vi "GetLimsTestsForBench.vi"(8 "error in (no error)":errorcluster, 9 "creation date":timestamp, 10 "workbench":string, 11 "ByteGSAPIBase in":refnum<class "ByteGSAPIBase.lvclass">) -> (0 "error out":errorcluster, 2 "list of tests":T1[](array[typedef]), 3 "ByteGSAPIBase out":refnum<class "ByteGSAPIBase.lvclass">)   [LabVIEW 2019, in "ByteGSWebAPI.lvlib" / "ByteGSAPIBase.lvclass"]
doc: "Request the list of Tests based on Workstation and Creation date (optional)"
uses:
  ByteGSAPIBase.lvclass
  TypeDef/Test.ctl
  TypeDef/Asset.ctl
  ByteGSAPIBase.lvclass/ByteGSAPIBase.ctl
  <vilib>/Bytelabs/ByteREST/ByteRESTClass/ByteRESTBase/RESTBase.lvclass
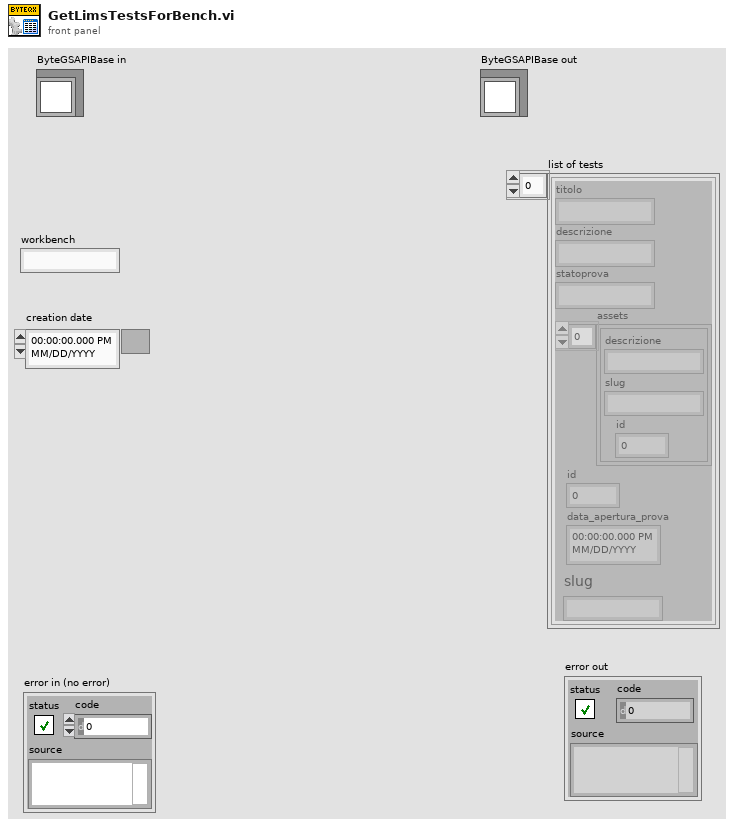
[diagram p1: front panel]
types:
  T1 = typedef "ByteGSWebAPI.lvlib/ByteGSAPIBase.lvclass/Test.ctl" = cluster{"titolo":string, "descrizione":string, "statoprova":string, "assets":T2[], "id":i32, "data_apertura_prova":timestamp, "slug":string}
  T2 = typedef "ByteGSWebAPI.lvlib/ByteGSAPIBase.lvclass/Asset.ctl" = cluster{"descrizione":string, "slug":string, "id":i32}
  T3 = cluster{"titolo":string, "descrizione":string, "statoprova":string, "assets":cluster{"descrizione":string, "slug":string, "id":i32}[], "data_apertura_prova":string, "id":i32, "slug":string}[]
  T4 = cluster{"descrizione":string, "slug":string, "id":i32}[]
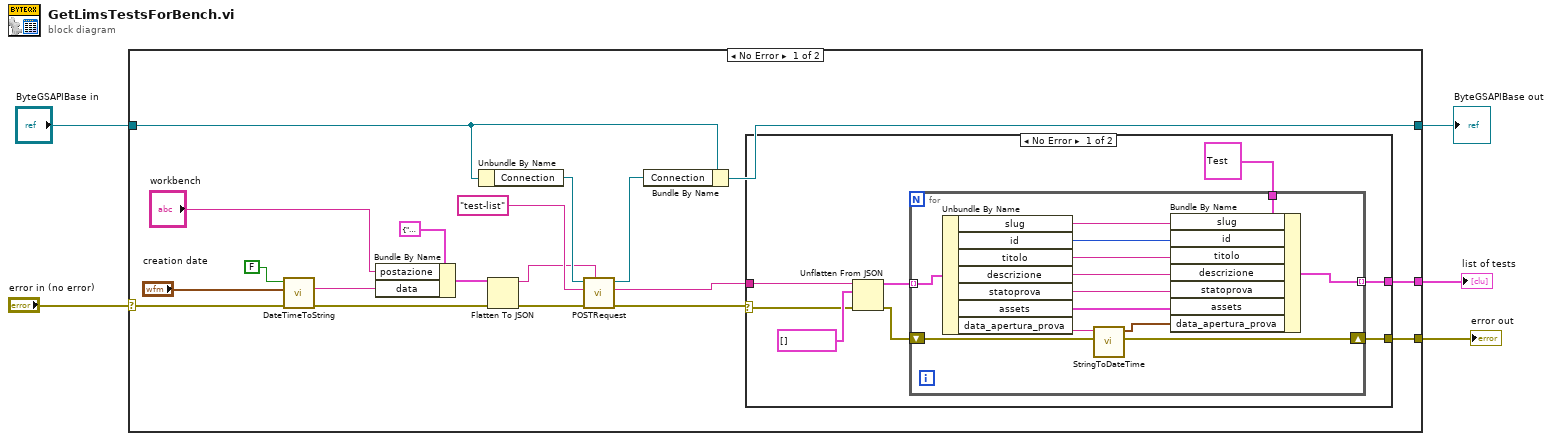
[diagram p0: block diagram]
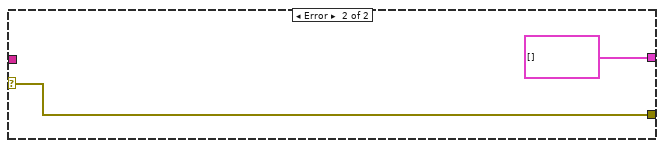
[diagram p2: hidden frame]
diagram:
  n1 = case shown="No Error" "error in (no error)" {
    selector: "error in (no error)" -> [w11 w49]
    tunnel: [w17 w49] -> w4
    tunnel: [w22 w48] -> w2
    tunnel: "ByteGSAPIBase in" -> [w15 w48]
    tunnel: [w16 _] -> w1
    frame No Error {
      n2 = call "DateTimeToString.vi"("error in"=w11, "current time"="creation date", "include Time?"=FALSE ("Time")) -> ("error out"=w12:errorcluster, "date string"=w10:string)  [unwired: 7 in]
      n3 = Bundle By Name(cluster=cluster{"postazione":string, "data":string} {"postazione"="", "data"=""} ("Request"), "postazione"="workbench", "data"=w10) -> (w13:cluster{"postazione":string, "data":string})
      n4 = Unbundle By Name(w15) -> ("Connection"=w24:refnum<class "RESTBase.lvclass">)
      n5 = Flatten To JSON(anything=w13, error in (no error)=w12) -> (JSON string=w20:string, 11:w19:errorcluster)  [unwired: 1 in]
      n6 = call-dynamic "POSTRequest.vi"("Body in"=w20, "error in (no error)"=w19, "Request"="test-list", "ByteRESTBase in"=w24) -> ("error out"=w7:errorcluster, "Body"=w18:string, "ByteRESTBase out"=w23:refnum<class "RESTBase.lvclass">)  [unwired: 4 in, 1 out]
      n7 = Bundle By Name(cluster=w15, "Connection"=w23) -> (w22:refnum<class "ByteGSAPIBase.lvclass">)
      n8 = case shown="No Error" w7 {
        selector: w7 -> [w25 w47]
        tunnel: w18 -> [w32 _]
        tunnel: [w28 w47] -> w17
        tunnel: [w27 T1[] []] -> w16
        frame No Error {
          n9 = Unflatten From JSON(JSON string=w32, type and defaults=T3 [], error in (no error)=w25) -> (value=w30:T3, error out=w29:errorcluster)  [unwired: 4 in]
          n10 = for {
            tunnel: w30 -> [w45] mode=indexing
            tunnel: T1 {"titolo"="", "descrizione"="", "statoprova"="", "assets"=[], "id"=0, "data_apertura_prova"=timestamp(0 s since 1904-01-01), "slug"=""} ("ByteGSWebAPI.lvlib:ByteGSAPIBase.lvclass:Test") -> [w44]
            shift-right: [w34] -> w28
            shift-left: w29 -> [w35]
            tunnel: [w38] -> w27 mode=indexing
            n11 = Unbundle By Name(w45) -> ("slug"=w33:string, "id"=w43:i32, "titolo"=w42:string, "descrizione"=w41:string, "statoprova"=w40:string, "assets"=w39:T4, "data_apertura_prova"=w37:string)
            n12 = call "StringToDateTime.vi"("error in (no error)"=w35, "datetime string"=w37) -> ("error out"=w34:errorcluster, "timestamp"=w36:timestamp)  [unwired: 8 in]
            n13 = Bundle By Name(cluster=w44, "slug"=w33, "id"=w43, "titolo"=w42, "descrizione"=w41, "statoprova"=w40, "assets"=w39, "data_apertura_prova"=w36) -> (w38:T1)
          }
        }
        frame Error {
        }
      }
    }
    frame Error {
    }
  }
  "error out" <- w4
  "ByteGSAPIBase out" <- w2
  "list of tests" <- w1
